vi "PracticeTank Controller.vi"() -> ()   [LabVIEW 2017]
uses:
  Tank State Machine Enum.ctl
panel:
  in  "Remote IO?":bool
  in  "Slide":dbl(slide) scale=0.0..30.0
  in  "stop":bool
  in  "Start":bool
  out "Tank":dbl(slide) scale=0.0..10.0
  in  "High Speed?":bool
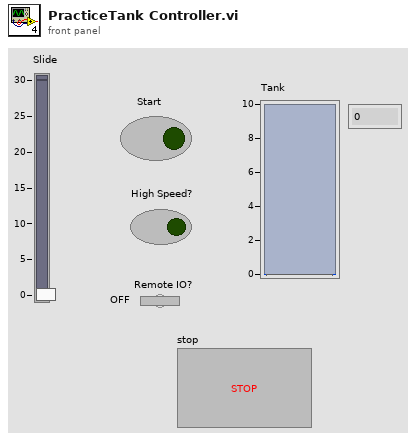
[diagram p1: front panel]
types:
  T1 = typedef "Tank State Machine Enum.ctl" = enum16{"idle", "fill", "tankFull"}
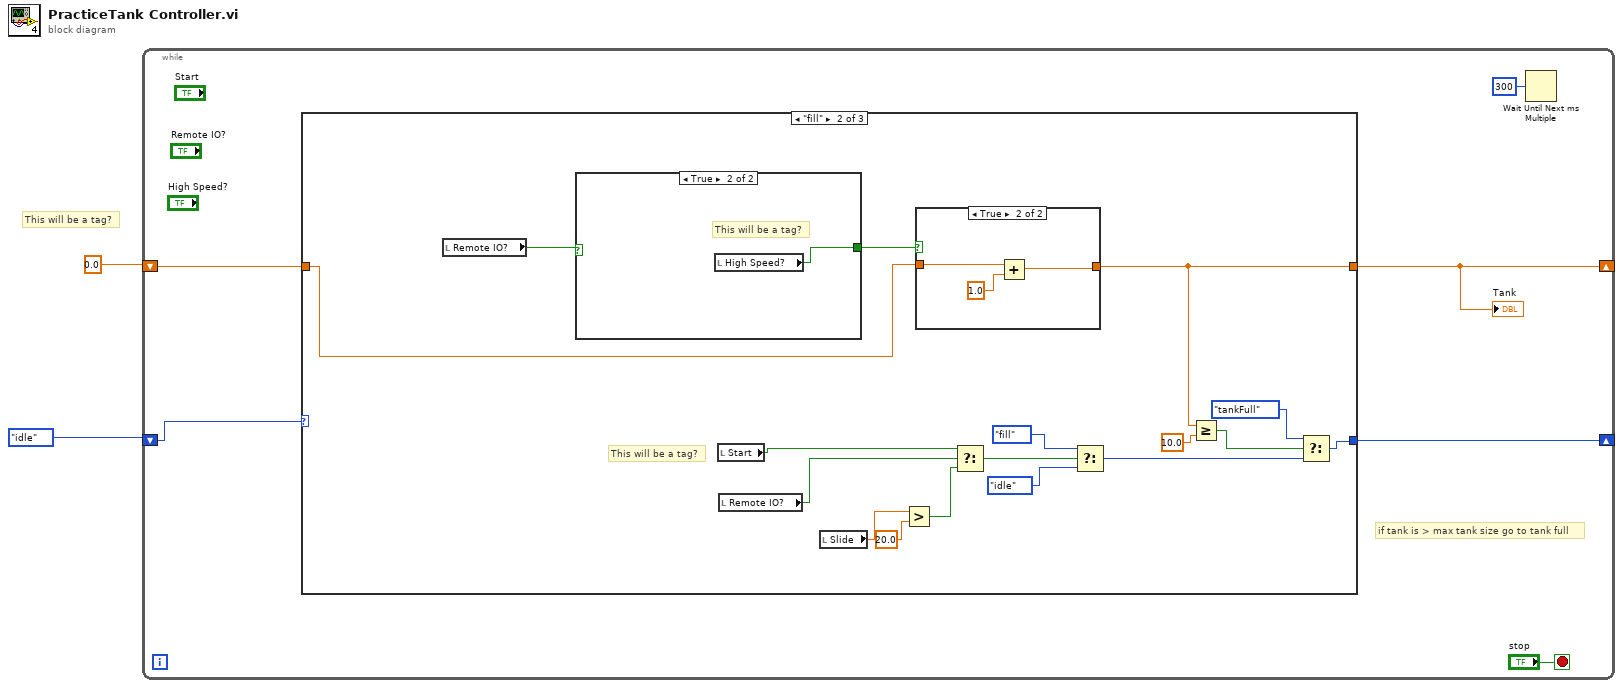
[diagram p0: block diagram]
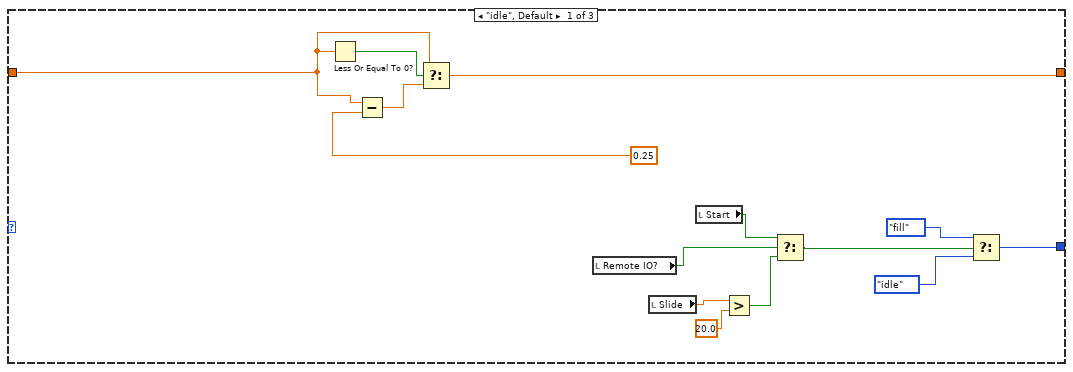
[diagram p2: hidden frame]
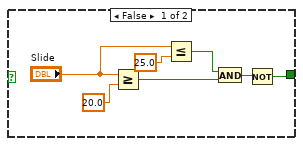
[diagram p3: hidden frame]
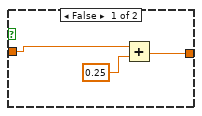
[diagram p4: hidden frame]
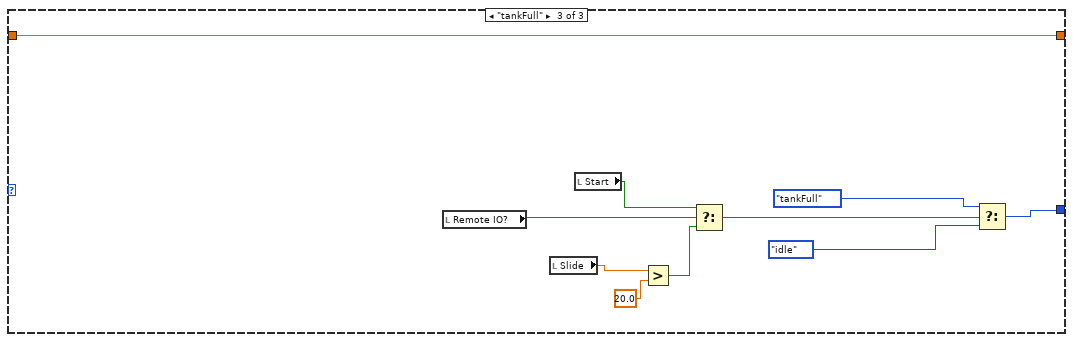
[diagram p5: hidden frame]
diagram:
  # "This will be a tag?"
  n1 = while {
    shift-right: [w3] -> _
    shift-left: Tank_State_Machine_Enum."idle" -> [w7]
    shift-right: [w4] -> _
    shift-left: 0.0 -> [w5]
    stop <- "stop" stop-if-true
    # "if tank is > max tank size go to tank full"
    n2 = case shown="\"fill\"" w7 {
      tunnel: w5 -> [w15 w30 w63]
      tunnel: [w17 w37 w63] -> w4
      tunnel: [w19 w33 w60] -> w3
      frame "idle", Default {
        n3 = Less Or Equal To 0?(x=w15) -> (x <= 0?=w16:bool)
        n4 = Subtract(x=w15, y=0.25) -> (x-y=w18:dbl)
        n5 = Select(t=w15, s=w16, f=w18) -> (s? t:f=w17:dbl)
        n6 = local read "Remote IO?"() -> (w9:bool)
        n7 = local read "Slide"() -> (w13:dbl)
        n8 = local read "Start"() -> (w12:bool)
        n9 = Greater?(x=w13, y=20.0) -> (0:w11:bool)
        n10 = Select(t=w12, s=w9, f=w11) -> (s? t:f=w10:bool)
        n11 = Select(t=Tank_State_Machine_Enum."fill", s=w10, f=Tank_State_Machine_Enum."idle") -> (s? t:f=w19:T1)
      }
      frame "fill" {
        # "This will be a tag?"
        n12 = local read "Remote IO?"() -> (w29:bool)
        n13 = case shown="True" w29 {
          tunnel: [w40 w47] -> w31
          frame False {
            n14 = Greater Or Equal?(x="Slide", y=20.0) -> (x >= y?=w43:bool)
            n15 = Less Or Equal?(x="Slide", y=25.0) -> (x <= y?=w42:bool)
            n16 = And(x=w42, y=w43) -> (x .and. y?=w41:bool)
            n17 = Not(x=w41) -> (.not. x?=w40:bool)
          }
          frame True {
            # "This will be a tag?"
            n18 = local read "High Speed?"() -> (w47:bool)
          }
        }
        n19 = local read "Start"() -> (w23:bool)
        n20 = local read "Remote IO?"() -> (w28:bool)
        n21 = local read "Slide"() -> (w24:dbl)
        n22 = Greater?(x=w24, y=20.0) -> (0:w26:bool)
        n23 = case shown="True" w31 {
          tunnel: [w49 w52] -> w37
          tunnel: w30 -> [w48 w51]
          frame False {
            n24 = Add(x=w48, y=0.25) -> (x+y=w49:dbl)
          }
          frame True {
            n25 = Add(x=w51, y=1.0) -> (x+y=w52:dbl)
          }
        }
        n26 = Select(t=w23, s=w28, f=w26) -> (s? t:f=w25:bool)
        n27 = Select(t=Tank_State_Machine_Enum."fill", s=w25, f=Tank_State_Machine_Enum."idle") -> (s? t:f=w32:T1)
        n28 = Greater Or Equal?(x=w37, y=10.0) -> (x >= y?=w36:bool)
        n29 = Select(t=Tank_State_Machine_Enum."tankFull", s=w36, f=w32) -> (s? t:f=w33:T1)
      }
      frame "tankFull" {
        n30 = local read "Remote IO?"() -> (w56:bool)
        n31 = local read "Slide"() -> (w55:dbl)
        n32 = local read "Start"() -> (w57:bool)
        n33 = Greater?(x=w55, y=20.0) -> (0:w58:bool)
        n34 = Select(t=w57, s=w56, f=w58) -> (s? t:f=w54:bool)
        n35 = Select(t=Tank_State_Machine_Enum."tankFull", s=w54, f=Tank_State_Machine_Enum."idle") -> (s? t:f=w60:T1)
      }
    }
    "Tank" <- w4
    n36 = Wait Until Next ms Multiple(millisecond multiple=u32 300) -> ()  [unwired: 1 out]
  }
